vi "Timer FG.vi"(8 "error in":errorcluster, 10 "Action":enum16{"set", "get"}(ring)) -> (0 "error out":errorcluster, 2 "Elapsed time (ms)":dbl)   [LabVIEW 2018]
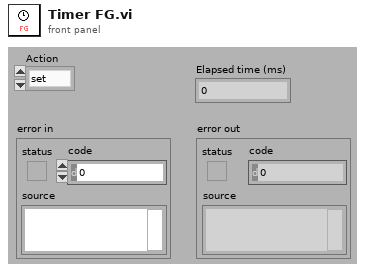
[diagram p1: front panel]
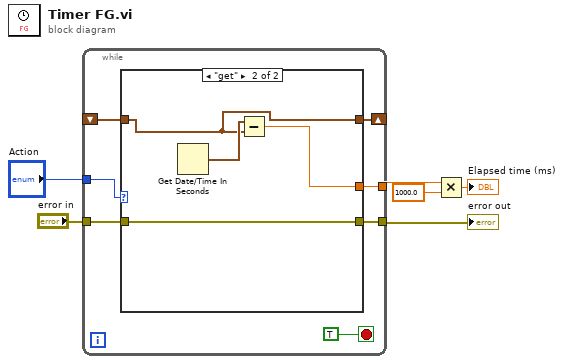
[diagram p0: block diagram]
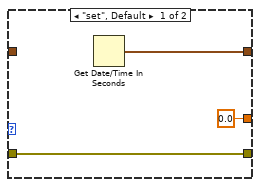
[diagram p2: hidden frame]
diagram:
  n1 = while {
    tunnel: [w12] -> w3
    tunnel: [w8] -> w6
    tunnel: "error in" -> [w7]
    tunnel: "Action" -> [w11]
    shift-right: [w10] -> _
    shift-left: _ -> [w9]
    stop <- TRUE ("stop") stop-if-true
    n2 = case shown="\"get\"" w11 {
      tunnel: [0.0 w20] -> w12
      tunnel: [w16 w18] -> w10
      tunnel: w9 -> [_ w18]
      tunnel: [w14 w17] -> w8
      tunnel: w7 -> [w14 w17]
      frame "set", Default {
        n3 = Get Date/Time In Seconds() -> (seconds since 1Jan1904=w16:timestamp)
      }
      frame "get" {
        n4 = Get Date/Time In Seconds() -> (seconds since 1Jan1904=w19:timestamp)
        n5 = Subtract(x=w19, y=w18) -> (x-y=w20:dbl)
      }
    }
  }
  "error out" <- w6
  n6 = Multiply(x=w3, y=1000.0) -> (x*y=→"Elapsed time (ms)":dbl)
